vi "MakeVIFrontMost.vi"(0 "VI Reference In":refnum<vi>, 11 "error in":errorcluster) -> (4 "VI Reference Out":refnum<vi>, 15 "error out":errorcluster)   [LabVIEW 2016, in "Drona.lvlib"]
doc: "Makes the front panel of the VI to frontmost, given the VI reference"
uses:
  Drona.lvlib
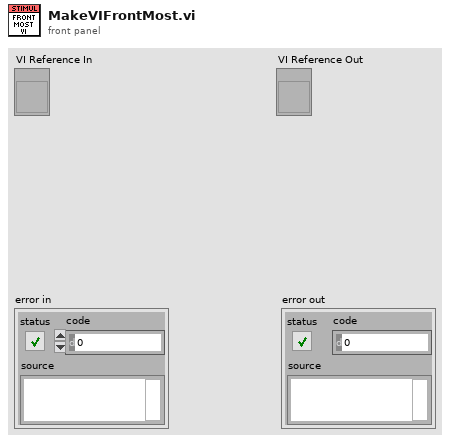
[diagram p1: front panel]
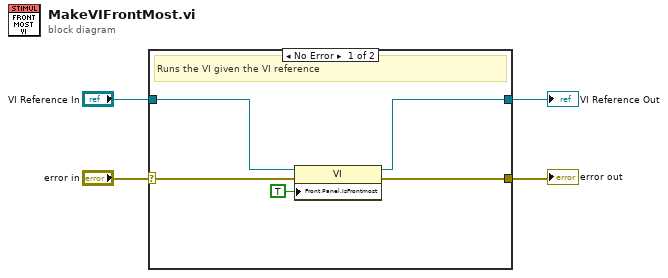
[diagram p0: block diagram]
diagram:
  n1 = case shown="No Error" "error in" {
    selector: "error in" -> [w9 w11]
    tunnel: "VI Reference In" -> [w6 w10]
    tunnel: [w7 w10] -> w2
    tunnel: [w8 w11] -> w1
    frame No Error {
      # "Runs the VI given the VI reference"
      n2 = property class="VI"(reference=w6, error in=w9, "Front Panel.IsFrontmost"=TRUE ("Front Panel Window:Is Frontmost")) -> (reference out=w7:refnum<vi>, error out=w8:errorcluster)
    }
    frame Error {
    }
  }
  "error out" <- w1
  "VI Reference Out" <- w2
